vi "Open Drive.vi"() -> (3 "Drive Motors":T1={"DevStatus"={"status"=FALSE, "code"=0, "source"=""}, "Motors[]"=[], "Square Inputs"=FALSE, "Max Output"=1.0})   [LabVIEW 2014]
uses:
  <vilib>/Rock Robotics/WPI/RobotDrive/WPI_RobotDriveDevRef.ctl
  <vilib>/Rock Robotics/WPI/MotorControl/WPI_MotorControlDeviceRef.ctl
  <vilib>/Rock Robotics/WPI/MotorControl/WPI_MotorControlType.ctl
  <vilib>/Rock Robotics/SystemInterfaces/Typedef/FPGA_TypedefDigitalModule.ctl
  <vilib>/Rock Robotics/SystemInterfaces/DIO/FPGA_DIOPWMChannel.ctl
  <vilib>/Rock Robotics/WPI/PWM/WPI_PWMDeadband.ctl
  <vilib>/Rock Robotics/WPI/CAN/Jaguar/SubVIs/WPI_CANJaguar_ControlMode.ctl
  <vilib>/Rock Robotics/WPI/CAN/TalonSRX/WPI_CANTalonSRX_APIControlMode.ctl
  <vilib>/Rock Robotics/WPI/PWM/WPI_PWMTransform_ConPane.ctl
  Robot Global Data.vi
  <vilib>/Rock Robotics/WPI/MotorControl/WPI_MotorControlOpenCANTalonSRX.vi
  <vilib>/Rock Robotics/WPI/RobotDrive/WPI_RobotDriveOpen4MotorWithExistingMotors.vi
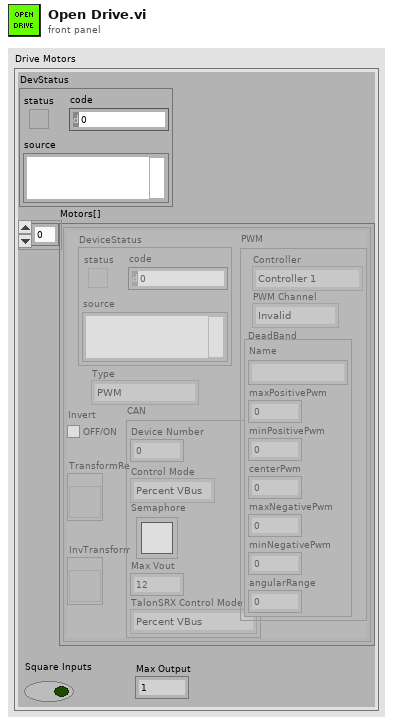
[diagram p1: front panel]
types:
  T1 = typedef "WPI_RobotDriveDevRef.ctl" = cluster{"DevStatus":errorcluster, "Motors[]":T2[], "Square Inputs":bool, "Max Output":dbl}
  T2 = typedef "WPI_MotorControlDeviceRef.ctl" = cluster{"DeviceStatus":errorcluster, "Type":T3, "PWM":cluster{"Controller":T4, "PWM Channel":T5, "DeadBand":T6}, "CAN":cluster{"Device Number":u8, "Control Mode":T7, "Semaphore":T8, "Max Vout":dbl, "TalonSRX Control Mode":T9}, "Invert":bool, "TransformRef":T10, "InvTransformRef":T10}
  T3 = typedef "WPI_MotorControlType.ctl" = enum16{"PWM", "CAN", "CANTalonSRX"}
  T4 = typedef "FPGA_TypedefDigitalModule.ctl" = enum16{"Controller 1"}
  T5 = typedef "FPGA_DIOPWMChannel.ctl" = enum8{"PWM 0", "PWM 1", "PWM 2", "PWM 3", "PWM 4", "PWM 5", "PWM 6", "PWM 7", "PWM 8", "PWM 9", "PWM MXP 0", "PWM MXP 1", "PWM MXP 2", "PWM MXP 3", "PWM MXP 4", "PWM MXP 5", "PWM MXP 6", "PWM MXP 7", "PWM MXP 8", "PWM MXP 9", "Invalid"}
  T6 = typedef "WPI_PWMDeadband.ctl" = cluster{"Name":string, "maxPositivePwm":i32, "minPositivePwm":i32, "centerPwm":i32, "maxNegativePwm":i32, "minNegativePwm":i32, "angularRange":u16}
  T7 = typedef "WPI_CANJaguar_ControlMode.ctl" = enum8{"Percent VBus", "Current", "Speed", "Position", "Voltage"}
  T8 = typedef "Semaphore RefNum" = refnum<k1>
  T9 = typedef "WPI_CANTalonSRX_APIControlMode.ctl" = enum8{"Percent VBus", "Speed", "Position", "Slave", "Unchanged / Invalid"}
  T10 = typedef "WPI_PWMTransform_ConPane.ctl" = refnum<vi>
  T11 = typedef "FPGA_DIOChannel.ctl" = enum8{"DIO 0", "DIO 1", "DIO 2", "DIO 3", "DIO 4", "DIO 5", "DIO 6", "DIO 7", "DIO 8", "DIO 9", "DIO MXP 0", "DIO MXP 1", "DIO MXP 2", "DIO MXP 3", "DIO MXP 4", "DIO MXP 5", "DIO MXP 6", "DIO MXP 7", "DIO MXP 8", "DIO MXP 9", "DIO MXP 10", "DIO MXP 11", "DIO MXP 12", "DIO MXP 13", "DIO MXP 14", "DIO MXP 15", "Invalid"}
  T12 = cluster{"Lift Motors":cluster{"Left Lift":dbl, "Right Lift":dbl}, "Sensors":cluster{"Limit Switches":cluster{"Bottom IR":T11, "Top IR":T11}, "Encoders":cluster{"Lift Encoder A Pin":T11, "Lift Encoder B Pin":T11}}, "Solenoids":cluster{"Left Clamp FWD":dbl, "Right Clamp FWD":dbl, "Brake":dbl, "Left Clamp BCK":dbl, "Right Clamp BCK":dbl, "Left Clamp PModule":dbl, "Right Clamp PModule":dbl, "Brake PModule":dbl}, "Drive Motors":cluster{"Rear Left Motor":dbl, "Rear Right Motor":dbl, "Front Left Motor":dbl, "Front Right Motor":dbl}}
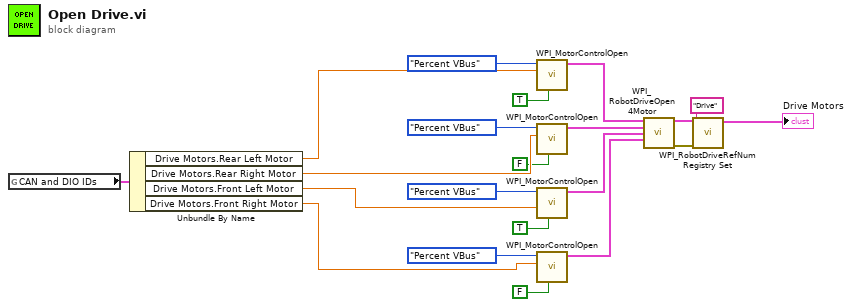
[diagram p0: block diagram]
diagram:
  n1 = global read "Robot Global Data.vi" "CAN and DIO IDs"() -> (w16:T12)
  n2 = Unbundle By Name(w16) -> ("Drive Motors.Rear Left Motor"=w12:dbl, "Drive Motors.Rear Right Motor"=w11:dbl, "Drive Motors.Front Left Motor"=w10:dbl, "Drive Motors.Front Right Motor"=w9:dbl)
  n3 = call-poly <vilib>:"WPI_MotorControlOpen.vi"("Invert"=TRUE, "Device Number"=w12, "Control Mode"=WPI_CANTalonSRX_APIControlMode."Percent VBus") -> ("MotorControlDeviceRef"=w21:T2)  [unwired: 7 in, 1 out]
  n4 = call-poly <vilib>:"WPI_MotorControlOpen.vi"("Invert"=FALSE, "Device Number"=w11, "Control Mode"=WPI_CANTalonSRX_APIControlMode."Percent VBus") -> ("MotorControlDeviceRef"=w20:T2)  [unwired: 7 in, 1 out]
  n5 = call-poly <vilib>:"WPI_MotorControlOpen.vi"("Invert"=TRUE, "Device Number"=w10, "Control Mode"=WPI_CANTalonSRX_APIControlMode."Percent VBus") -> ("MotorControlDeviceRef"=w19:T2)  [unwired: 7 in, 1 out]
  n6 = call-poly <vilib>:"WPI_MotorControlOpen.vi"("Invert"=FALSE, "Device Number"=w9, "Control Mode"=WPI_CANTalonSRX_APIControlMode."Percent VBus") -> ("MotorControlDeviceRef"=w18:T2)  [unwired: 7 in, 1 out]
  n7 = call-poly <vilib>:"WPI_RobotDriveOpen4Motor.vi"("Rear Left Motor Dev Ref"=w21, "Rear Right Motor Dev Ref"=w20, "Front Left Motor Dev Ref"=w19, "Front Right Motor Dev Ref"=w18) -> ("RobotDriveDevRef"=w3:T1, "error out"=w4:errorcluster)  [unwired: 10 in]
  n8 = call <vilib>:"WPI_RobotDriveRefNum Registry Set.vi"("error in (no error)"=w4, "refnum name"="Drive", "RobotDriveDevRef"=w3) -> ("RobotDriveDevRef"=→"Drive Motors":T1)  [unwired: 7 in, 1 out]
